vi "Enable Axes.vi"(8 "error in":errorcluster, 10 "axis names":string[](array[string])=["X", "Y", "Z", "U"], 11 "Gantry in":refnum<class "Gantry.lvclass">) -> (0 "error out":errorcluster, 3 "Gantry out":refnum<class "Gantry.lvclass">)   [LabVIEW 2026, in "Gantry.lvclass"]
uses:
  Gantry.lvclass
  <instrlib>/Aerotech Automation1/Aerotech Automation1.lvlib
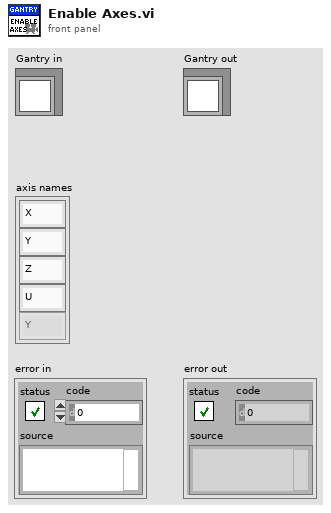
[diagram p1: front panel]
types:
  T1 = typedef "Virtual Modes.ctl" = enum16{"Nonvirtual", "Virtual"}
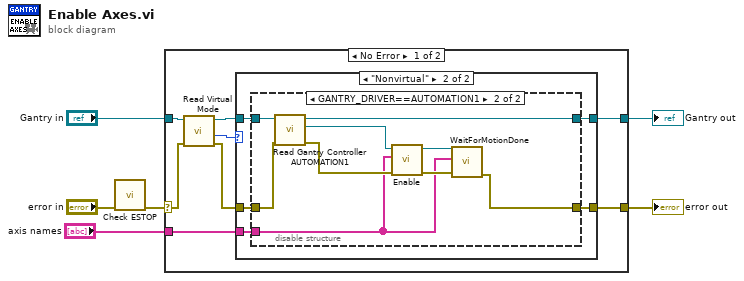
[diagram p0: block diagram]
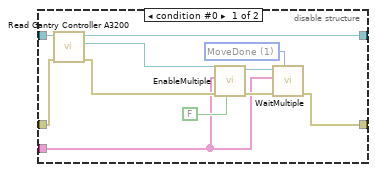
[diagram p3: hidden frame]
diagram:
  n1 = call "Check ESTOP.vi"("error in"="error in") -> ("error out"=w3:errorcluster)  [unwired: 10 in]
  n2 = case shown="No Error" w3 {
    selector: w3 -> [w9 w43]
    tunnel: [w14 w43] -> w6
    tunnel: [w13 w42] -> w5
    tunnel: "Gantry in" -> [w12 w42]
    tunnel: "axis names" -> [w7 _]
    frame No Error {
      n3 = call-dynamic "Read Virtual Mode.vi"("error in (no error)"=w9, "Gantry in"=w12) -> ("error out"=w8:errorcluster, "Virtual Mode"=w10:T1, "Gantry out"=w11:refnum<class "Gantry.lvclass">)  [unwired: 6 in, 1 out]
      n4 = case shown="\"Nonvirtual\"" w10 {
        tunnel: w8 -> [w15 w19]
        tunnel: [w15 w21] -> w14
        tunnel: w11 -> [w16 w20]
        tunnel: [w16 w18] -> w13
        tunnel: w7 -> [_ w17]
        frame "Virtual" {
        }
        frame "Nonvirtual" {
          n5 = disable-structure shown="GANTRY_DRIVER==AUTOMATION1" {
            disable-tunnel: [w28 w33] -> w21
            disable-tunnel: w20 -> [w27 w35]
            disable-tunnel: w19 -> [w26 w36]
            disable-tunnel: [w24 w34] -> w18
            disable-tunnel: w17 -> [w22 w37]
            frame condition #0 {
              w30 = 1 items=["InPosition", "MoveDone"] ("wait option?")
              n6 = call "Read Gantry Controller A3200.vi"("error in (no error)"=w26, "Gantry in"=w27) -> ("error out"=w25:errorcluster, "A3200 controller out"=w23:refnum<k24>, "Gantry out"=w24:refnum<class "Gantry.lvclass">)  [unwired: 7 in]
              n7 = call "EnableMultiple.vi"("return immediately"=FALSE, "error in (no error)"=w25, "axis names"=w22, "controller in"=w23) -> ("error out"=w29:errorcluster, "controller out"=w31:refnum<k24>)  [unwired: 6 in]
              n8 = call "WaitMultiple.vi"("wait option?"=w30, "error in (no error)"=w29, "axis names"=w22, "controller in"=w31) -> ("error out"=w28:errorcluster)  [unwired: 5 in, 2 out]
            }
            frame condition #1 (active) {
              n9 = call "Read Gantry Controller AUTOMATION1.vi"("error in (no error)"=w36, "Gantry in"=w35) -> ("error out"=w41:errorcluster, "Controller AUTOMATION1"=w40:refnum<k24>, "Gantry out"=w34:refnum<class "Gantry.lvclass">)  [unwired: 7 in]
              n10 = call <instrlib>:"Enable.vi"("error in (no error)"=w41, "axes"=w37, "Controller Refnum"=w40) -> ("error out"=w38:errorcluster, "Controller Refnum out"=w39:refnum<k24>)  [unwired: 7 in]
              n11 = call <instrlib>:"WaitForMotionDone.vi"("error in (no error)"=w38, "axes"=w37, "Controller Refnum"=w39) -> ("error out"=w33:errorcluster)  [unwired: 7 in, 1 out]
            }
          }
        }
      }
    }
    frame Error {
    }
  }
  "error out" <- w6
  "Gantry out" <- w5
